vi "Test MQTT-3.12.4-1.vi"(8 "error in (no error)":errorcluster, 11 "Connection Config":refnum<class "Connection.lvclass">) -> (0 "error out":errorcluster, 3 "Connection Config dup":refnum<class "Connection.lvclass">)   [LabVIEW 2013]
uses:
  <vilib>/LabVIEW Open Source Project/MQTT Connection/MQTT_Connection/Connection/Connection.lvclass
  <vilib>/addons/_JKI Toolkits/Caraya/classes/Test/Test.lvclass
  <vilib>/LabVIEW Open Source Project/MQTT Client/Client class/Client.lvclass
  <vilib>/addons/_JKI Toolkits/Caraya/classes/Assert/Assert.lvclass
  <vilib>/LabVIEW Open Source Project/MQTT Connection/MQTT_Base/Base Class/MQTT_Base.lvclass
panel:
  out "ping time (ms)":i32
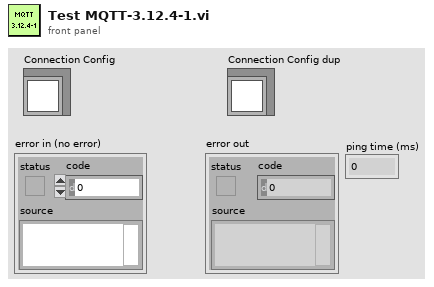
[diagram p1: front panel]
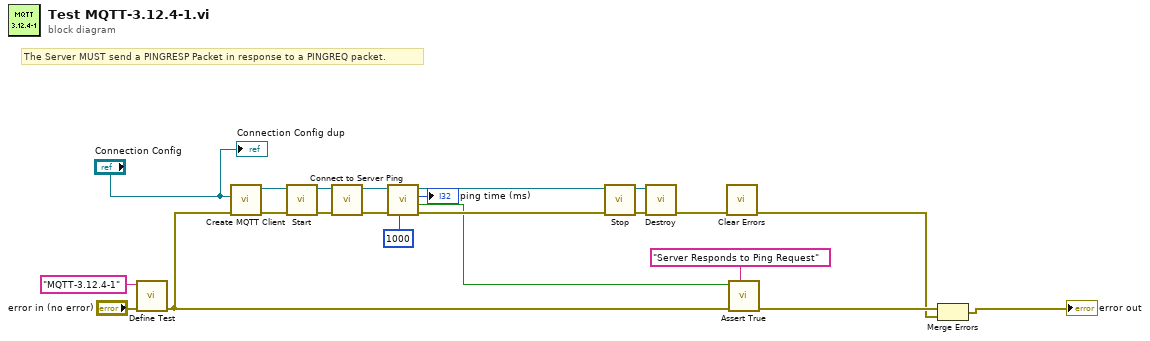
[diagram p0: block diagram]
diagram:
  # "The Server MUST send a PINGRESP Packet in response to a PINGREQ packet."
  n1 = call <vilib>:"Define Test.vi"("error in (no error)"="error in (no error)", "Label (VI Title)"="MQTT-3.12.4-1") -> ("error out"=w10:errorcluster)  [unwired: 9 in]
  n2 = call <vilib>:"Create MQTT Client.vi"("error in (no error)"=w10, "Connection Configuration"="Connection Config") -> ("error out"=w14:errorcluster, "Client out"=w15:refnum<class "Client.lvclass">)  [unwired: 8 in]
  n3 = call <vilib>:"Start.vi"("error in (no error)"=w14, "MQTT_Base in"=w15) -> ("error out"=w18:errorcluster, "MQTT_Base out"=w19:refnum<class "Client.lvclass">)  [unwired: 7 in, 1 out]
  n4 = call <vilib>:"Connect to Server.vi"("error in (no error)"=w18, "Client in"=w19) -> ("error out"=w8:errorcluster, "Client out"=w9:refnum<class "Client.lvclass">)  [unwired: 6 in, 2 out]
  n5 = call <vilib>:"Ping.vi"("timeout (1000 ms)"=1000, "error in (no error)"=w8, "Client in"=w9) -> ("error out"=w7:errorcluster, "Server responded"=w4:bool, "ping time"=→"ping time (ms)":i32, "Client out"=w5:refnum<class "Client.lvclass">)  [unwired: 5 in]
  n6 = call <vilib>:"Stop.vi"("error in (no error)"=w7, "MQTT_Base in"=w5) -> ("error out"=w16:errorcluster, "MQTT_Base out"=w17:refnum<class "Client.lvclass">)  [unwired: 7 in, 1 out]
  n7 = call <vilib>:"Destroy.vi"("error in (no error)"=w16, "MQTT_Base in"=w17) -> ("error out"=w12:errorcluster)  [unwired: 8 in, 1 out]
  n8 = call <vilib>:"Clear Errors.vi"("error in (no error)"=w12) -> ("error out"=w1:errorcluster)  [unwired: 6 in]
  n9 = call <vilib>:"Assert True.vi"("Label"="Server Responds to Ping Request", "error in (no error)"=w10, "True?"=w4) -> ("error out"=w11:errorcluster)  [unwired: 8 in]
  n10 = Merge Errors(w11, w1) -> (→"error out":errorcluster)
  "Connection Config dup" <- "Connection Config"
